vi "get_all_output_status.vi"(8 "error in (no error)":errorcluster, 11 "VISA resource name":refnum<visa-resource-name>) -> (0 "error out":errorcluster, 2 "Output active array":bool[](array[boolean]), 3 "VISA resource name out":refnum<visa-resource-name>)   [LabVIEW 2018, in "Inficon IC6.lvlib"]
doc: "Query the status of all outputs."
uses:
  <instrlib>/Inficon IC6/Inficon IC6.lvlib
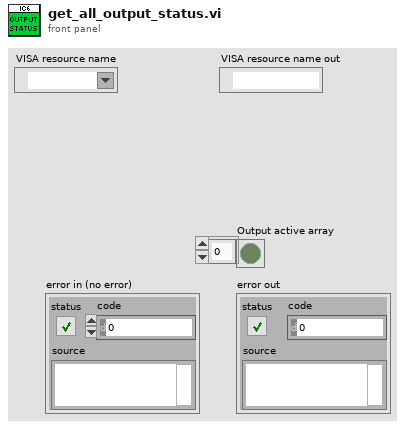
[diagram p1: front panel]
types:
  T1 = enum16{"Source", "General", "Input name", "Process name", "Logic", "Material", "Material name", "Output name", "Process", "Sensor", "Output type", "User message", "Layer", ""}
  T2 = enum16{"Hello", "Query", "Remote action", "Status", "Update"}
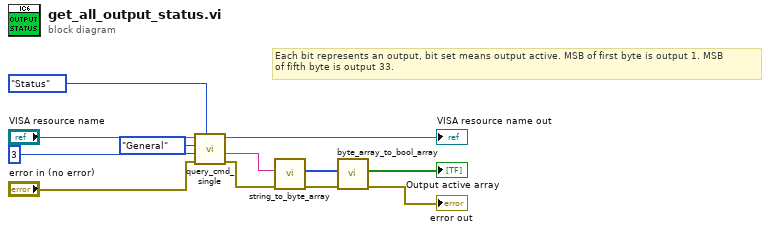
[diagram p0: block diagram]
diagram:
  # "Each bit represents an output, bit set means output active. MSB of first byte is output 1. MSB\nof fifth byte is output 33."
  n1 = call <instrlib>:"query_cmd_single.vi"("Command group"=T2."Status", "error in (no error)"="error in (no error)", "Command ID"=u8 3, "Command subgroup"=T1."General", "VISA resource name"="VISA resource name") -> ("error out"=w6:errorcluster, "formatted response"=w7:string, "VISA resource name out"=→"VISA resource name out":refnum<visa-resource-name>)  [unwired: 2 in, 2 out]
  n2 = call <instrlib>:"string_to_byte_array.vi"("error in (no error)"=w6, "Byte"=w7) -> ("error out"=w5:errorcluster, "Int array"=w3:u8[])  [unwired: 8 in]
  n3 = call <instrlib>:"byte_array_to_bool_array.vi"("error in (no error)"=w5, "Byte array"=w3) -> ("error out"=→"error out":errorcluster, "Boolean array"=→"Output active array":bool[])  [unwired: 8 in]
